vi "GE 5565PIORC.Registers.DMADPR0.Direction of Transfer.Set.vi"(8 "error in (no error)":errorcluster, 10 "Transfer Direction":enum16{"Host to RFM", "RFM to Host"}(ring), 11 "GE 5565PIORC in":refnum<class "GE 5565PIORC.lvclass">) -> (0 "error out":errorcluster, 3 "GE 5565PIORC out":refnum<class "GE 5565PIORC.lvclass">)   [LabVIEW 2017, in "GE 5565PIORC.lvclass"]
doc: "Writing a one (1) indicates transfer from the RFM to the PCI bus. Writing a zero (0) indicates transfer from the PCI bus to the RFM."
uses:
  GE 5565PIORC.lvclass
  GE 5565PIORC.Registers.Local Configuration.ctl
  GE 5565PIORC.lvclass/GE 5565PIORC.ctl
  GE 5565PIORC.Registers.Local Configuration.Read (U32).vi
  GE 5565PIORC.Registers.Local Configuration.Write (U32).vi
  Methods/GE 5565PIORC.Bit Manipulation.Set Bit (U32).vi
  Methods/GE 5565PIORC.Registers.Read.vi
  Methods/GE 5565PIORC.Registers.Read (U32).vi
  Methods/GE 5565PIORC.Registers.Write.vi
  Methods/GE 5565PIORC.Registers.Write (U32).vi
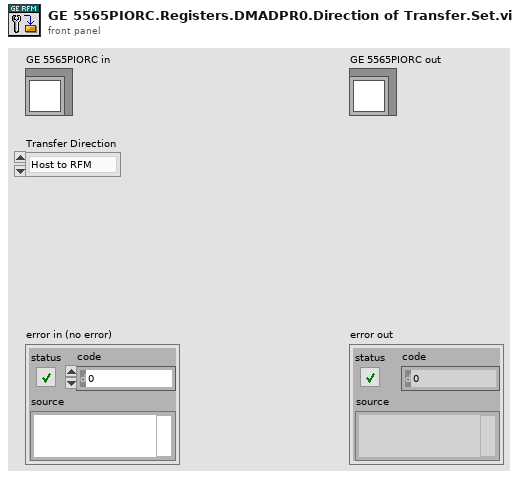
[diagram p1: front panel]
types:
  T1 = typedef "GE 5565PIORC.lvclass/GE 5565PIORC.Registers.Local Configuration.ctl" = u32
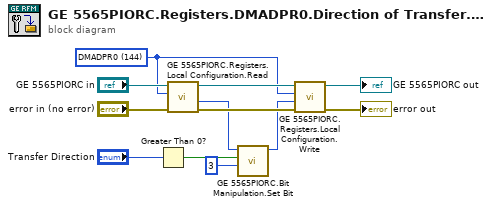
[diagram p0: block diagram]
diagram:
  w6 = T1 144 items=["MARBR"=8, "BIGEND"=12, "INTCSR"=104, "PCIHREV"=116, "DMAMODE0"=128, "DMAPADR0"=132, "DMALADR0"=136, "DMASIZ0"=140, "DMADPR0"=144, "DMACSR0"=168, "DMADAC0"=180, "LAS1RR"=240, "LAS1BA"=244] ("Local Configuration Registers")
  n1 = Greater Than 0?(x="Transfer Direction") -> (x > 0?=w2:bool)
  n2 = call-poly "GE 5565PIORC.Registers.Local Configuration.Read.vi"("error in (no error)"="error in (no error)", "Register"=w6, "GE 5565PIORC in"="GE 5565PIORC in") -> ("error out"=w12:errorcluster, "Value"=w5:u32, "GE 5565PIORC out"=w9:refnum<class "GE 5565PIORC.lvclass">)  [unwired: 6 in]
  n3 = call-poly "GE 5565PIORC.Bit Manipulation.Set Bit.vi"("bit index"=3, "bit"=w2, "packed value in"=w5) -> ("packed value out"=w4:u32)  [unwired: 8 in]
  n4 = call-poly "GE 5565PIORC.Registers.Local Configuration.Write.vi"("error in (no error)"=w12, "Value"=w4, "Register"=w6, "GE 5565PIORC in"=w9) -> ("error out"=→"error out":errorcluster, "GE 5565PIORC out"=→"GE 5565PIORC out":refnum<class "GE 5565PIORC.lvclass">)  [unwired: 6 in]
